vi "Format Version for Display.vi"(11 "Strings":string[](array[string])) -> (1 "Latest Vers":string[](array[string]), 2 "Displayed String":string, 3 "String":string)   [LabVIEW 2020, in "LMH-LINX.lvlib"]
uses:
  <vilib>/MakerHub/LINX/LMH-LINX.lvlib
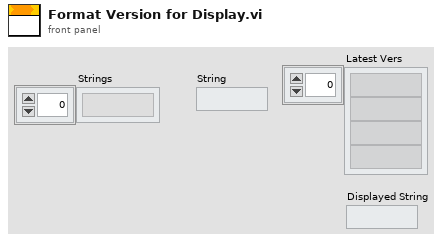
[diagram p1: front panel]
types:
  T1 = cluster{"Substrings":string[], "token string":string}
  T2 = cluster{"Substrings":string[], "token string":string}[]
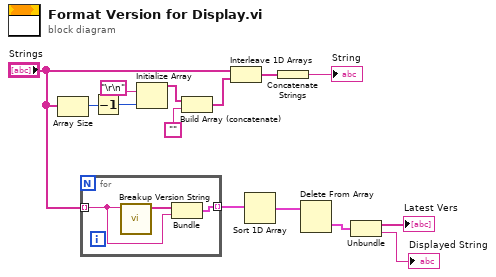
[diagram p0: block diagram]
diagram:
  n1 = Array Size(array="Strings") -> (size(s)=w8:i32)
  n2 = for {
    tunnel: "Strings" -> [w15] mode=indexing
    tunnel: [w16] -> w5 mode=indexing
    n3 = call <vilib>:"Breakup Version String.vi"("Vers String"=w15) -> ("Substrings"=w17:string[])  [unwired: 10 in]
    n4 = Bundle("Substrings"=w17, "token string"=w15) -> (w16:T1)  [unwired: 1 in]
  }
  n5 = Decrement(x=w8) -> (x-1=w9:i32)
  n6 = Initialize Array("\r\n", w9) -> (w13:string[])
  n7 = Build Array (concatenate)(w13, "") -> (w14:string[])
  n8 = Interleave 1D Arrays("Strings", w14) -> (w10:string[])
  n9 = Sort 1D Array(array=w5) -> (sorted array=w4:T2)
  n10 = Concatenate Strings(w10) -> (→"String":string)
  n11 = Delete From Array(array=w4) -> (deleted portion=w3:T1)  [unwired: 2 in, 1 out]
  n12 = Unbundle(w3) -> ("Substrings"=→"Latest Vers":string[], "token string"=→"Displayed String":string)
